vi "Pressure to Caller.vi"(8 "error in (no error)":errorcluster, 10 "Analog Input Waveform":waveform(dbl), 11 "Pressure to Caller in":refnum<class "Pressure to Caller.lvclass">) -> (0 "error out":errorcluster)   [LabVIEW 2021, in "Pressure to Caller.lvclass"]
uses:
  Pressure to Caller.lvclass
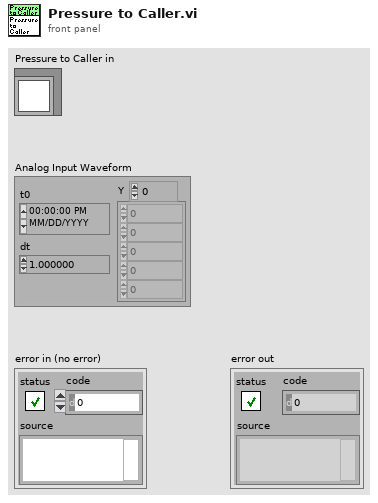
[diagram p1: front panel]
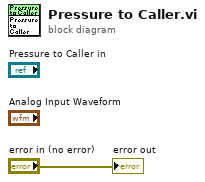
[diagram p0: block diagram]
diagram:
  "error out" <- "error in (no error)"
